vi "BuildMATRIX.vi"(7 "Data Type":T1=enum."miMATRIX", 8 "data":dbl[](array[numeric]), 10 "byte order":T2(ring)=enum."little-endian", 11 "String in":string) -> (3 "String out":string)   [LabVIEW 2022 SP3]
uses:
  miDataType.ctl
panel:
  out "length":i32
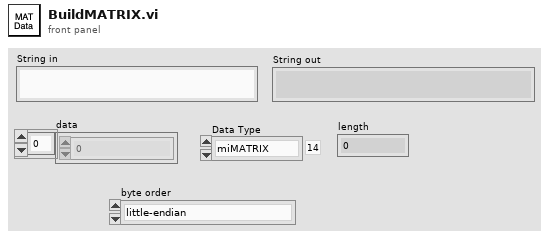
[diagram p1: front panel]
types:
  T1 = typedef "miDataType.ctl" = enum16{"illegal", "miINT8", "miUINT8", "miINT16", "miUINT16", "miINT32", "miUINT32", "miSINGLE", "--", "miDOUBLE", "---", "----", "miINT64", "miUINT64", "miMATRIX", "miCOMPRESSED", "miUTF8", "miUTF16", "miUTF32", "udefined"}
  T2 = enum16{"big-endian, network order", "native, host order", "little-endian"}
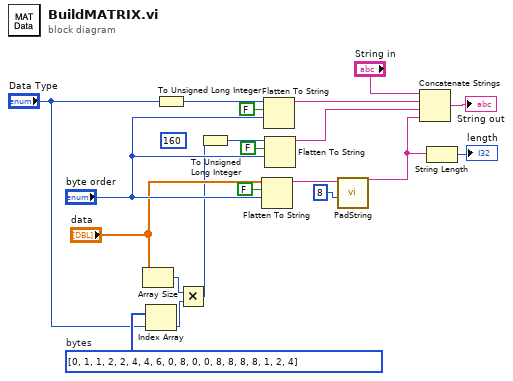
[diagram p0: block diagram]
diagram:
  (unwired) u32 160 ("number")
  w10 = i32[] [0, 1, 1, 2, 2, 4, 4, 6, 0, 8, 0, 0, 8, 8, 8, 8, 1, 2, 4]  # bytes
  n1 = Array Size(array="data") -> (size(s)=w9:i32)
  n2 = Index Array(array=w10, index="Data Type") -> (element=w8:i32)
  n3 = To Unsigned Long Integer(number="Data Type") -> (unsigned 32bit integer=w15:u32)
  n4 = Multiply(x=w9, y=w8) -> (x*y=w2:i32)
  n5 = To Unsigned Long Integer(number=w2) -> (unsigned 32bit integer=w16:u32)
  n6 = Flatten To String(anything="data", prepend array or string size? (T)=FALSE, byte order (0:big-endian, network order)="byte order") -> (data string=w6:string)  [unwired: 1 in, 2 out]
  n7 = Flatten To String(anything=w15, prepend array or string size? (T)=FALSE, byte order (0:big-endian, network order)="byte order") -> (data string=w19:string)  [unwired: 1 in, 2 out]
  n8 = Flatten To String(anything=w16, prepend array or string size? (T)=FALSE, byte order (0:big-endian, network order)="byte order") -> (data string=w20:string)  [unwired: 1 in, 2 out]
  n9 = call "PadString.vi"("size"=8, "data"=w6) -> ("String"=w5:string)  [unwired: 9 in]
  n10 = Concatenate Strings("String in", w19, w20, w5) -> (→"String out":string)
  n11 = String Length(string=w5) -> (length=→"length":i32)
